vi "Configure Waveform Modulation State.vi"(7 "Enable Modulated Output (T: Enable)":bool=TRUE, 8 "error in (no error)":errorcluster, 10 "Waveform Generator Number (1: Waveform Generator 1)":i32(ring)=1 items=["Waveform Generator 1"=1], 11 "VISA resource name":refnum<visa-resource-name>) -> (0 "error out":errorcluster, 3 "VISA resource name out":refnum<visa-resource-name>)   [LabVIEW 2017, in "Agilent 2000 3000 X-Series.lvlib"]
doc: "Enables or disables modulated waveform generator output. You can enable modulation for all waveform generator function types except pulse, DC, and noise."
uses:
  Agilent 2000 3000 X-Series.lvlib
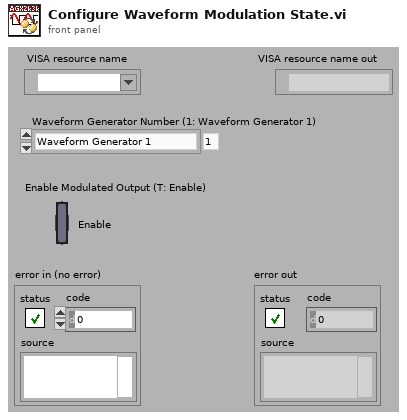
[diagram p1: front panel]
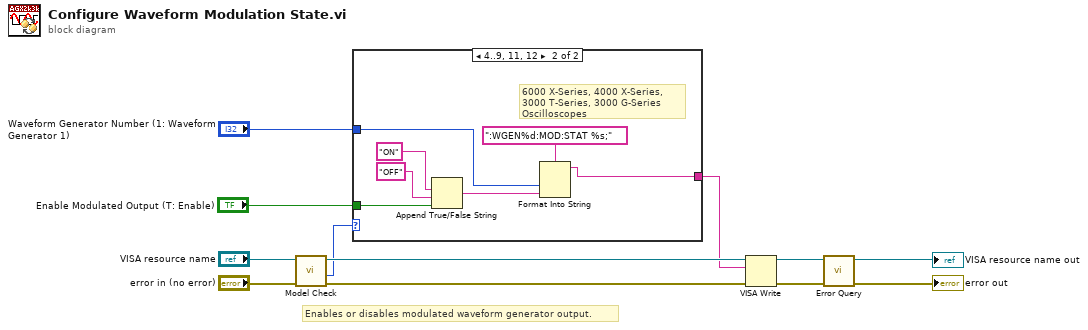
[diagram p0: block diagram]
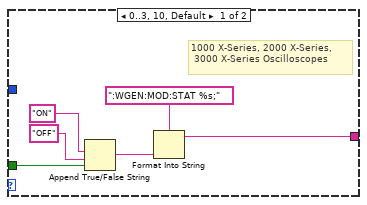
[diagram p2: hidden frame]
diagram:
  # "Enables or disables modulated waveform generator output."
  n1 = call "Model Check.vi"("error in (no error)"="error in (no error)", "VISA resource name"="VISA resource name") -> ("error out"=w7:errorcluster, "Model"=w2:i32, "VISA resource name out"=w8:refnum<visa-resource-name>)  [unwired: 7 out]
  n2 = case shown="4..9, 11, 12" w2 {
    tunnel: "Enable Modulated Output (T: Enable)" -> [w14 w21]
    tunnel: "Waveform Generator Number (1: Waveform Generator 1)" -> [_ w20]
    tunnel: [w13 w19] -> w1
    frame 0..3, 10, Default {
      # "1000 X-Series, 2000 X-Series,\n 3000 X-Series Oscilloscopes"
      n3 = Append True/False String(1:w14, 2:"OFF", 3:"ON") -> (0:w16:string)  [unwired: 1 out]
      n4 = Format Into String(format string=":WGEN:MOD:STAT %s;", w16) -> (resulting string=w13:string)  [unwired: 2 in, 1 out]
    }
    frame 4..9, 11, 12 {
      # "6000 X-Series, 4000 X-Series, 3000 T-Series, 3000 G-Series Oscilloscopes"
      n5 = Append True/False String(1:w21, 2:"OFF", 3:"ON") -> (0:w22:string)  [unwired: 1 out]
      n6 = Format Into String(format string=":WGEN%d:MOD:STAT %s;", w20, w22) -> (resulting string=w19:string)  [unwired: 2 in, 1 out]
    }
  }
  n7 = VISA Write(VISA resource name=w8, write buffer=w1, error in (no error)=w7) -> (VISA resource name out=w6:refnum<visa-resource-name>, error out=w5:errorcluster)  [unwired: 1 out]
  n8 = call "Error Query.vi"("error in (no error)"=w5, "VISA resource name"=w6) -> ("error out"=→"error out":errorcluster, "VISA resource name out"=→"VISA resource name out":refnum<visa-resource-name>)  [unwired: 6 in, 2 out]
